vi "load dark symbol set.vi"(8 "error in (no error)":errorcluster, 11 "tree reference":refnum<vi>) -> (0 "error out":errorcluster, 3 "tree reference":refnum<vi>)   [LabVIEW 2020, in "UI_ItemSelect_OpenSource.lvlib"]
uses:
  UI_ItemSelect_OpenSource.lvlib
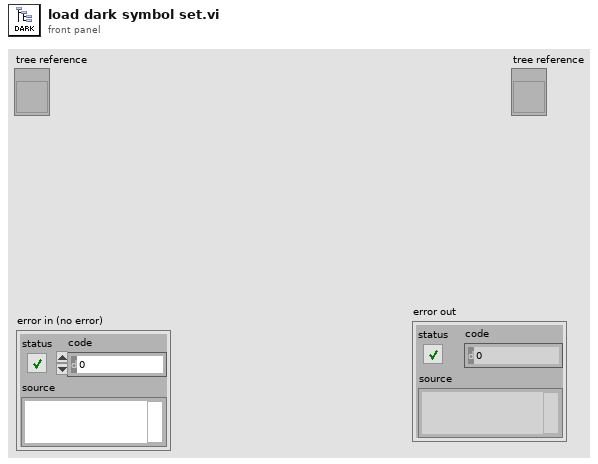
[diagram p1: front panel]
types:
  T1 = typedef "imagedata.ctl" = cluster{"image type":i32, "image depth":i32, "image":u8[], "mask":u8[], "colors":u32[], "Rectangle":cluster{"left":i16, "top":i16, "right":i16, "bottom":i16}}
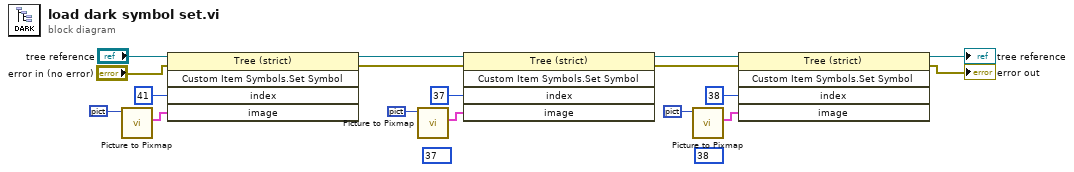
[diagram p0: block diagram]
diagram:
  (unwired) 38
  (unwired) 37
  n1 = call <vilib>:"Picture to Pixmap.vi"("picture"=picture bytes[291] ("Picture 3")) -> ("image data"=w16:T1)  [unwired: 9 in, 1 out]
  n2 = invoke class="Tree (strict)" method="Custom Item Symbols.Set Symbol"(reference="tree reference", error in="error in (no error)", "index"=41 ("Index"), "image"=w16) -> (reference out=w10:refnum<vi>, error out=w3:errorcluster)  [unwired: 1 in, 3 out]
  n3 = call <vilib>:"Picture to Pixmap.vi"("picture"=picture bytes[291] ("Picture 3")) -> ("image data"=w15:T1)  [unwired: 9 in, 1 out]
  n4 = invoke class="Tree (strict)" method="Custom Item Symbols.Set Symbol"(reference=w10, error in=w3, "index"=37 ("Index"), "image"=w15) -> (reference out=w11:refnum<vi>, error out=w2:errorcluster)  [unwired: 1 in, 3 out]
  n5 = call <vilib>:"Picture to Pixmap.vi"("picture"=picture bytes[291] ("Picture 3")) -> ("image data"=w12:T1)  [unwired: 9 in, 1 out]
  n6 = invoke class="Tree (strict)" method="Custom Item Symbols.Set Symbol"(reference=w11, error in=w2, "index"=38 ("Index"), "image"=w12) -> (reference out=→"tree reference":refnum<vi>, error out=→"error out":errorcluster)  [unwired: 1 in, 3 out]
